vi "AutoSequencer.vi"(0 "Auto Error In":errorcluster, 1 "Drive Advance In":bool, 2 "Drive Step In":i32, 4 "Manipulator Advance In":bool, 5 "Manipulator Step In":i32, 8 "Reinit Sequencer":bool) -> (14 "Auto Error Out":errorcluster, 15 "Drive Advance Out":bool, 16 "Drive Step Out":i32, 18 "Manipulator Advance Out":bool, 19 "Manipulator Step Out":i32)   [LabVIEW 2019]
doc: "This VI manages the autonomous sequence. The drive base and manipulator sequencers operate in parallel. Autonomous plays are written as text files and uploaded to the roboRIO via FileZilla. The appropriate play is slected prior to the match via the FRC 4265 Dashboard. For each sequencer, each step is composed of a command and a parameter string of arbitrary length. The drive sequencer selects commands using a case structure while the subsystem sequencer selects commands using static VI references (this disparate choice is made due to conflicting memory handling and ease-of-creation tradeoffs). Error checking and handling is supported. An autonomous test mode (for simulating autonomous plays on the robot cart) is supported. Status updates are sent to the FRC Driver Station and the FRC 4265 Dashboard throughout autonomous. Note that the autonomous sequencer may be also active during the begining of TeleOperated mode, as determined by the MasterRobotModeController.vi."
uses:
  sensors.vi
  constants.vi
  dsdata.vi
  autoninfo.vi
  3b074430-bbfe-494f-99f2-72c3d74da684.vi
  a18db1b9-ed6f-48db-83ed-89b9a31e5ef5.vi
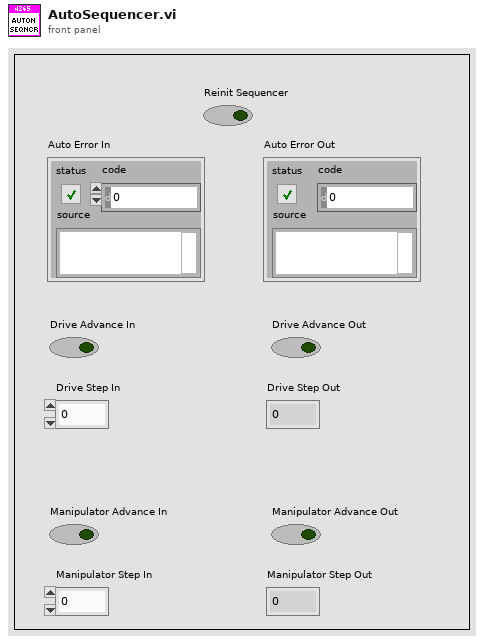
[diagram p1: front panel]
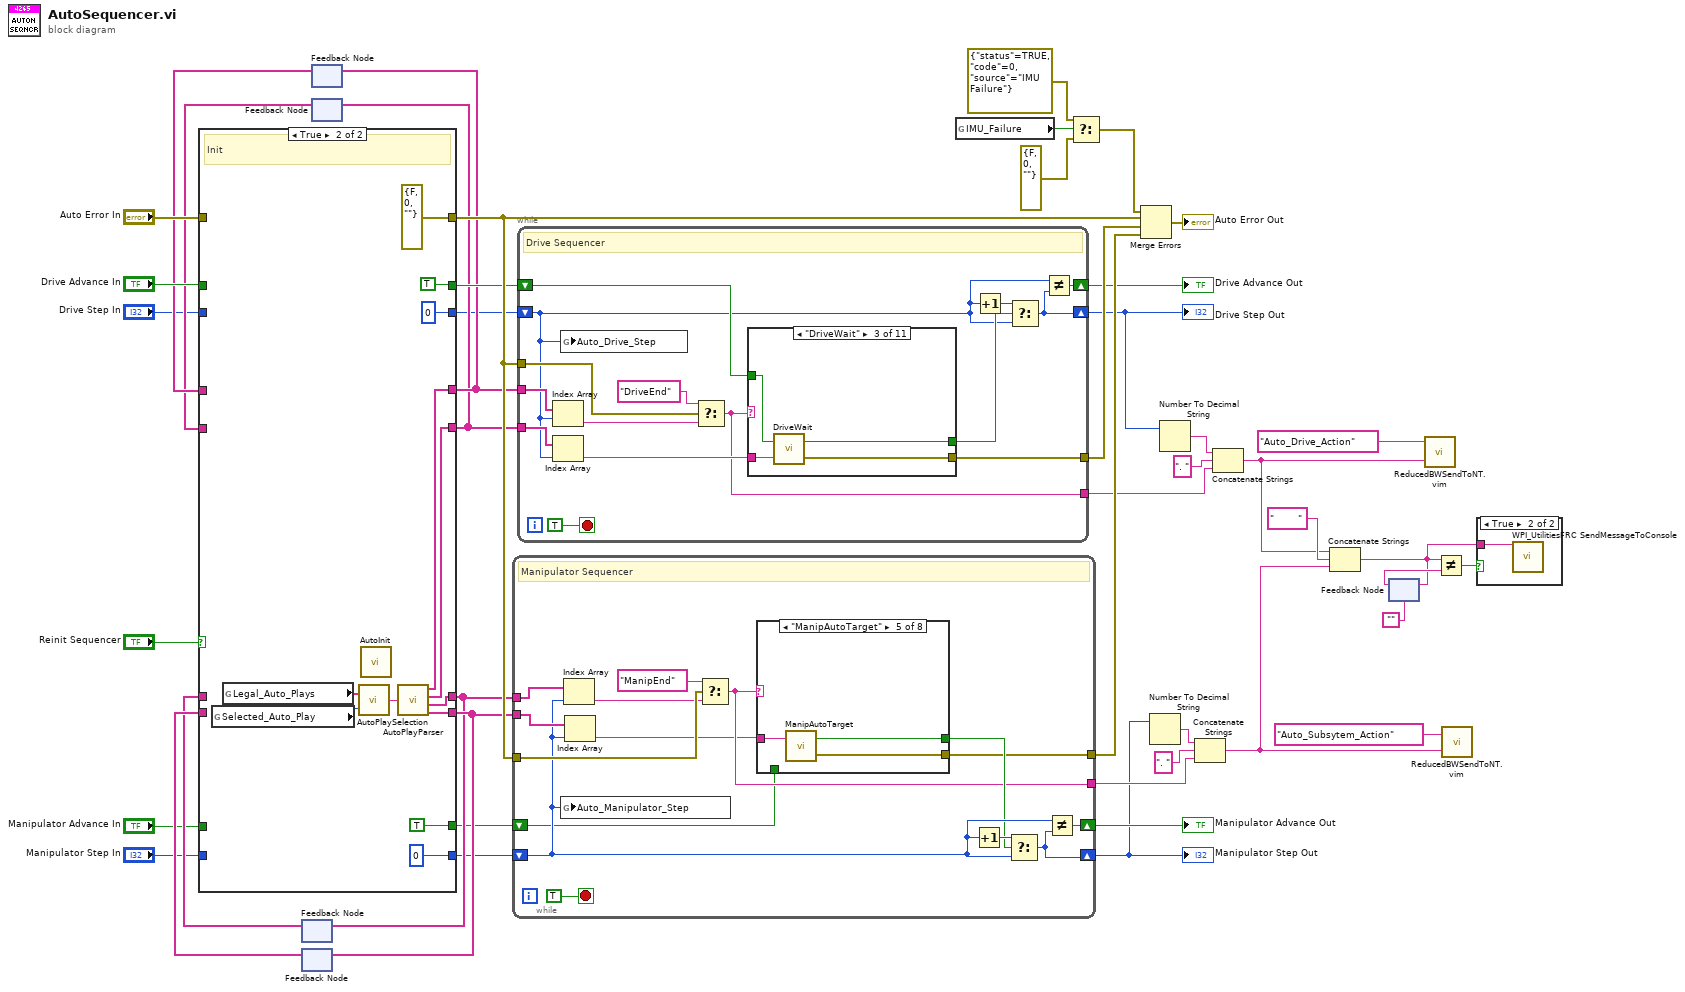
[diagram p0: block diagram]
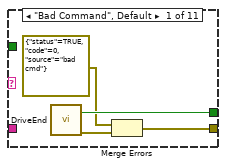
[diagram p3: hidden frame]
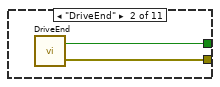
[diagram p4: hidden frame]
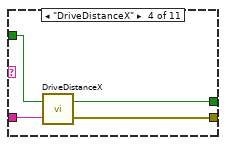
[diagram p5: hidden frame]
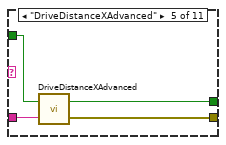
[diagram p6: hidden frame]
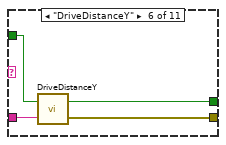
[diagram p7: hidden frame]
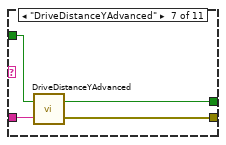
[diagram p8: hidden frame]
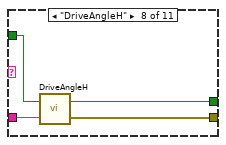
[diagram p9: hidden frame]
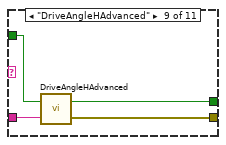
[diagram p10: hidden frame]
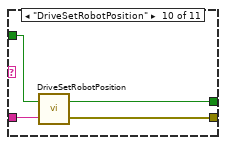
[diagram p11: hidden frame]
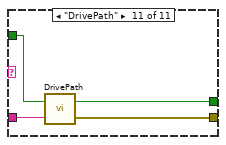
[diagram p12: hidden frame]
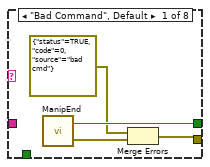
[diagram p14: hidden frame]
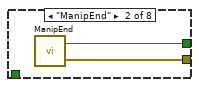
[diagram p15: hidden frame]
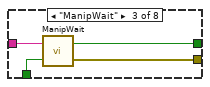
[diagram p16: hidden frame]
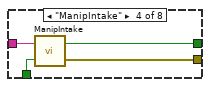
[diagram p17: hidden frame]
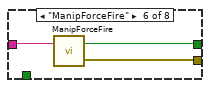
[diagram p18: hidden frame]
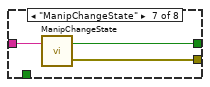
[diagram p19: hidden frame]
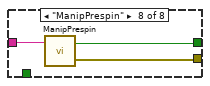
[diagram p20: hidden frame]
diagram:
  n1 = feedback #1() -> (w30:string[])  [unwired: 1 in]
  n2 = feedback #2() -> (w31:string[])  [unwired: 1 in]
  n3 = feedback #3() -> (w37:string[])  [unwired: 1 in]
  n4 = feedback #4() -> (w36:string[])  [unwired: 1 in]
  n5 = case shown="True" "Reinit Sequencer" {
    tunnel: "Manipulator Step In" -> [w53 _]
    tunnel: "Manipulator Advance In" -> [w54 _]
    tunnel: [w54 TRUE ("Advance Trigger")] -> w12
    tunnel: [w53 0] -> w26
    tunnel: [w52 w60] -> w28
    tunnel: [w51 w64] -> w29
    tunnel: w30 -> [w52 _]
    tunnel: w31 -> [w51 _]
    tunnel: [w50 0] -> w32
    tunnel: "Drive Step In" -> [w50 _]
    tunnel: [w49 w62] -> w34
    tunnel: [w48 w61] -> w35
    tunnel: w36 -> [w49 _]
    tunnel: w37 -> [w48 _]
    tunnel: [w47 TRUE] -> w38
    tunnel: "Drive Advance In" -> [w47 _]
    tunnel: [w46 errorcluster {"status"=FALSE, "code"=0, "source"=""} ("error constant")] -> w44
    tunnel: "Auto Error In" -> [w46 _]
    frame False {
      # "Pass"
    }
    frame True {
      # "Init"
      n6 = global read "dsdata.vi" "Selected_Auto_Play"() -> (w58:u16)
      n7 = global read "constants.vi" "Legal_Auto_Plays"() -> (w57:string[])
      n8 = call "AutoPlaySelection.vi"("Selected Auto Play"=w58, "Auto Plays"=w57) -> ("Autonomous Commands"=w56:string)
      n9 = call "AutoInit.vi"() -> ()  [unwired: 1 in]
      n10 = call "AutoPlayParser.vi"("Auto Play"=w56) -> ("Drive Command Strings"=w61:string[], "Drive Parameter Strings"=w62:string[], "Manipulator Command Strings"=w60:string[], "Manipulator Parameter Strings"=w64:string[])
    }
  }
  n11 = feedback-in #1(w28) -> ()
  n12 = feedback-in #2(w29) -> ()
  n13 = feedback-in #3(w35) -> ()
  n14 = feedback-in #4(w34) -> ()
  n15 = while {
    tunnel: w28 -> [w77]
    shift-right: [w79] -> w11
    shift-left: w26 -> [w73]
    shift-right: [w78] -> w23
    shift-left: w12 -> [w68]
    tunnel: w29 -> [w76]
    tunnel: [w70] -> w17
    tunnel: [w71] -> w45
    tunnel: w44 -> [w74]
    stop <- TRUE stop-if-true
    # "Manipulator Sequencer"
    n16 = global write "autoninfo.vi" "Auto_Manipulator_Step"(w73) -> ()
    n17 = Index Array(array=w77, index=w73) -> (element=w67:string)
    n18 = Index Array(array=w76, index=w73) -> (element=w69:string)
    n19 = Select(t="ManipEnd", s=w74, f=w67) -> (s? t:f=w70:string)
    n20 = case shown="\"ManipAutoTarget\"" w70 {
      tunnel: w69 -> [_ _ w91 w95 w98 w101 w104 w107]
      tunnel: [w85 w87 w90 w94 w97 w100 w103 w106] -> w72
      tunnel: [w83 w86 w89 w93 w96 w99 w102 w105] -> w71
      tunnel: w68 -> [_ _ w88 w92 _ _ _ _]
      frame "Bad Command", Default {
        n21 = call "ManipEnd.vi"() -> ("Error Out"=w84:errorcluster, "Advance Trigger"=w85:bool)  [unwired: 2 in]
        n22 = Merge Errors(errorcluster {"status"=TRUE, "code"=0, "source"="bad cmd"} ("Path Follow Error"), w84) -> (w83:errorcluster)
      }
      frame "ManipEnd" {
        n23 = call "ManipEnd.vi"() -> ("Error Out"=w86:errorcluster, "Advance Trigger"=w87:bool)  [unwired: 2 in]
      }
      frame "ManipWait" {
        n24 = call "ManipWait.vi"("Reinit"=w88, "Instruction String"=w91) -> ("Error Out"=w89:errorcluster, "Advance Trigger"=w90:bool)
      }
      frame "ManipIntake" {
        n25 = call "ManipIntake.vi"("Reinit"=w92, "Instruction String"=w95) -> ("Error Out"=w93:errorcluster, "Advance Trigger"=w94:bool)
      }
      frame "ManipAutoTarget" {
        n26 = call "ManipAutoTarget.vi"("Instruction String"=w98) -> ("Error Out"=w96:errorcluster, "Advance Trigger"=w97:bool)  [unwired: 1 in]
      }
      frame "ManipForceFire" {
        n27 = call "ManipForceFire.vi"("Instruction String"=w101) -> ("Error Out"=w99:errorcluster, "Advance Trigger"=w100:bool)  [unwired: 1 in]
      }
      frame "ManipChangeState" {
        n28 = call "ManipChangeState.vi"("Instruction String"=w104) -> ("Error Out"=w102:errorcluster, "Advance Trigger"=w103:bool)  [unwired: 1 in]
      }
      frame "ManipPrespin" {
        n29 = call "ManipPrespin.vi"("Instruction String"=w107) -> ("Error Out"=w105:errorcluster, "Advance Trigger"=w106:bool)  [unwired: 1 in]
      }
    }
    n30 = Increment(x=w73) -> (x+1=w81:i32)
    n31 = Select(t=w81, s=w72, f=w73) -> (s? t:f=w79:i32)
    n32 = Not Equal?(x=w73, y=w79) -> (x != y?=w78:bool)
  }
  "Manipulator Step Out" <- w11
  "Manipulator Advance Out" <- w23
  n33 = while {
    shift-right: [w117] -> w10
    shift-left: w32 -> [w108]
    tunnel: w35 -> [w120]
    tunnel: w34 -> [w119]
    shift-right: [w116] -> w39
    shift-left: w38 -> [w115]
    tunnel: [w109] -> w22
    tunnel: w44 -> [w113]
    tunnel: [w110] -> w43
    stop <- TRUE stop-if-true
    # "Drive Sequencer"
    n34 = Index Array(array=w120, index=w108) -> (element=w112:string)
    n35 = Index Array(array=w119, index=w108) -> (element=w118:string)
    n36 = global write "autoninfo.vi" "Auto_Drive_Step"(w108) -> ()
    n37 = Select(t="DriveEnd", s=w113, f=w112) -> (s? t:f=w109:string)
    n38 = case shown="\"DriveWait\"" w109 {
      tunnel: w118 -> [_ _ w130 w135 w139 w142 w147 w150 w155 w159 w163]
      tunnel: [w126 w128 w132 w134 w138 w144 w146 w152 w154 w160 w161] -> w114
      tunnel: w115 -> [_ _ w131 w136 w140 w143 w148 w151 w156 w158 w164]
      tunnel: [w124 w127 w129 w133 w137 w141 w145 w149 w153 w157 w162] -> w110
      frame "Bad Command", Default {
        n39 = call "DriveEnd.vi"() -> ("Error Out"=w125:errorcluster, "Advance Trigger"=w126:bool)  [unwired: 2 in]
        n40 = Merge Errors(errorcluster {"status"=TRUE, "code"=0, "source"="bad cmd"} ("Path Follow Error"), w125) -> (w124:errorcluster)
      }
      frame "DriveEnd" {
        n41 = call "DriveEnd.vi"() -> ("Error Out"=w127:errorcluster, "Advance Trigger"=w128:bool)  [unwired: 2 in]
      }
      frame "DriveWait" {
        n42 = call "DriveWait.vi"("Parameter String"=w130, "Reinit"=w131) -> ("Error Out"=w129:errorcluster, "Increment"=w132:bool)
      }
      frame "DriveDistanceX" {
        n43 = call "DriveDistanceX.vi"("Parameter String"=w135, "Reinit"=w136) -> ("Error Out"=w133:errorcluster, "Increment"=w134:bool)
      }
      frame "DriveDistanceXAdvanced" {
        n44 = call "DriveDistanceXAdvanced.vi"("Parameter String"=w139, "Reinit"=w140) -> ("Error Out"=w137:errorcluster, "Increment"=w138:bool)
      }
      frame "DriveDistanceY" {
        n45 = call "DriveDistanceY.vi"("Parameter String"=w142, "Reinit"=w143) -> ("Error Out"=w141:errorcluster, "Increment"=w144:bool)
      }
      frame "DriveDistanceYAdvanced" {
        n46 = call "DriveDistanceYAdvanced.vi"("Parameter String"=w147, "Reinit"=w148) -> ("Error Out"=w145:errorcluster, "Increment"=w146:bool)
      }
      frame "DriveAngleH" {
        n47 = call "DriveAngleH.vi"("Parameter String"=w150, "Reinit"=w151) -> ("Error Out"=w149:errorcluster, "Increment"=w152:bool)
      }
      frame "DriveAngleHAdvanced" {
        n48 = call "DriveAngleHAdvanced.vi"("Parameter String"=w155, "Reinit"=w156) -> ("Error Out"=w153:errorcluster, "Increment"=w154:bool)
      }
      frame "DriveSetRobotPosition" {
        n49 = call "DriveSetRobotPosition.vi"("Parameter String"=w159, "Reinit"=w158) -> ("Error Out"=w157:errorcluster, "Increment"=w160:bool)
      }
      frame "DrivePath" {
        n50 = call "DrivePath.vi"("Parameter String"=w163, "Reinit"=w164) -> ("Path Follower Error"=w162:errorcluster, "Increment"=w161:bool)
      }
    }
    n51 = Increment(x=w108) -> (x+1=w121:i32)
    n52 = Select(t=w121, s=w114, f=w108) -> (s? t:f=w117:i32)
    n53 = Not Equal?(x=w108, y=w117) -> (x != y?=w116:bool)
  }
  "Drive Advance Out" <- w39
  "Drive Step Out" <- w10
  n54 = global read "sensors.vi" "IMU_Failure"() -> (w16:bool)
  n55 = Select(t=errorcluster {"status"=TRUE, "code"=0, "source"="IMU Failure"} ("error constant"), s=w16, f=errorcluster {"status"=FALSE, "code"=0, "source"=""} ("error constant")) -> (s? t:f=w13:errorcluster)
  n56 = Merge Errors(w13, w44, w43, w45) -> (→"Auto Error Out":errorcluster)
  n57 = Number To Decimal String(number=w11) -> (decimal integer string=w18:string)  [unwired: 1 in]
  n58 = Number To Decimal String(number=w10) -> (decimal integer string=w20:string)  [unwired: 1 in]
  n59 = Concatenate Strings(w18, ". " ("string"), w17) -> (w5:string)
  n60 = Concatenate Strings(w20, ". " ("string"), w22) -> (w7:string)
  n61 = Concatenate Strings(w7, "        " ("string"), w5) -> (w1:string)
  n62 = feedback-in #5(w1) -> ()
  n63 = feedback #5("") -> (w4:string)
  n64 = call "ReducedBWSendToNT.vim"("Value In"=w7, "NT Name"="Auto_Drive_Action" ("Name")) -> ()  [unwired: 1 out]
  n65 = Not Equal?(x=w1, y=w4) -> (x != y?=w2:bool)
  n66 = call "ReducedBWSendToNT.vim"("Value In"=w5, "NT Name"="Auto_Subsytem_Action" ("Name")) -> ()  [unwired: 1 out]
  n67 = case shown="True" w2 {
    tunnel: w1 -> [_ w165]
    frame False {
    }
    frame True {
      n68 = call <vilib>:"WPI_UtilitiesFRC SendMessageToConsole.vi"("Message"=w165) -> ()  [unwired: 14 in, 1 out]
    }
  }
